vi "Test1_Network Connectivity.vi"(8 "error in":errorcluster, 10 "command line":string="ping -n 2 127.0.0.1", 11 "Sequence Context In":refnum<k7>) -> (0 "error out":errorcluster, 3 "Return Packets(%)":i32=100)   [LabVIEW 2021]
doc: "You can use the System Exec VI to call command line utilities that return standard output to the command shell. You also can call interactive applications that you intend to launch using System Exec, but interact with using the UI of the executable."
uses:
  <vilib>/regexp/Match Regular Expression.xnode
panel:
  out "standard output":string="\r\nPinging 127.0.0.1 with 32 bytes of data:\r\nReply from 127.0.0.1: bytes=32 time<1ms TTL=128\r\nReply from 127.0.0.1: bytes=32 time<1ms TTL=128\r\n\r\nPing statistics for 127.0.0.1:\r\n    Packets: Sent = 2, Received = 2, Lost = 0 (0% loss),\r\nApproximate round trip times in milli-seconds:\r\n    Minimum = 0ms, Maximum = 0ms, Average = 0ms\r\n"
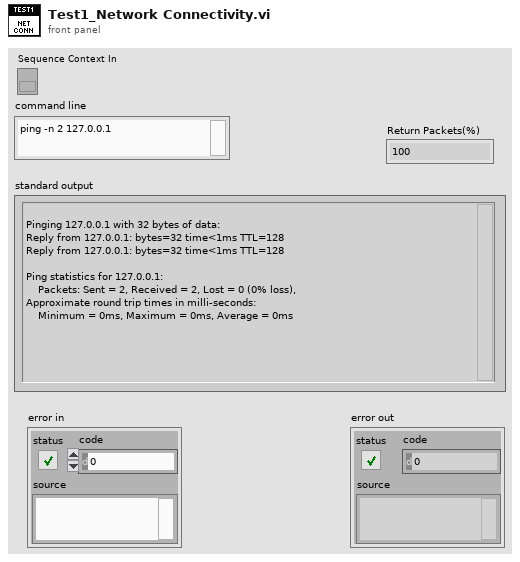
[diagram p1: front panel]
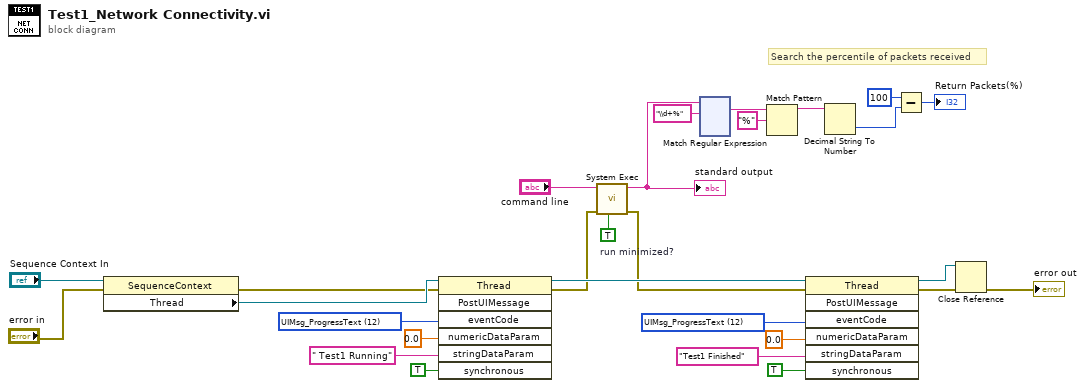
[diagram p0: block diagram]
diagram:
  w7 = 12 items=["UIMsg_BreakOnUserRequest"=1, "UIMsg_BreakOnBreakpoint"=2, "UIMsg_BreakOnRunTimeError"=3, "UIMsg_Trace"=4, "UIMsg_TerminatingExecution"=5, "UIMsg_AbortingExecution"=6, "UIMsg_KillingExecutionThreads"=7, "UIMsg_EndExecution"=8, "UIMsg_ShutDownComplete"=9, "UIMsg_StartExecution"=10, "UIMsg_ProgressPercent"=11, "UIMsg_ProgressText"=12, "UIMsg_StartInteractiveExecution"=13, "UIMsg_EndInteractiveExecution"=14, "UIMsg_TerminatingInteractiveExecution"=15, "UIMsg_TerminationCancelled"=16, "UIMsg_ResumeFromBreak"=17, "UIMsg_StartFileExecution"=18, "UIMsg_EndFileExecution"=19, "UIMsg_ShutDownCancelled"=20, "UIMsg_LocalizationSettingChanged"=21, "UIMsg_OpenWindows"=22, "UIMsg_TileWindows"=23, "UIMsg_CascadeWindows"=24, "UIMsg_ReportChanged"=25, "UIMsg_CloseWindows"=26, "UIMsg_RefreshWindows"=27, "UIMsg_ClientFileChanged"=28, "UIMsg_DisplayReport"=29, "UIMsg_ModelState_Initializing"=30, "UIMsg_ModelState_Waiting"=31, "UIMsg_ModelState_Identified"=32, "UIMsg_ModelState_BeginTesting"=33, "UIMsg_ModelState_TestingComplete"=34, "UIMsg_ModelState_PostProcessingComplete"=35, "UIMsg_ModelState_EnabledStateSet"=36, "UIMsg_ReportLocationChanged"=37, "UIMsg_GotoLocation"=38, "UIMsg_PushUndoItem"=39, "UIMsg_OutputMessages"=40, "UIMsg_TypePaletteFileListChanged"=41, "UIMsg_NonTerminatableThreadsArePreventingTermination"=42, "UIMsg_ModelState_PostProcessing"=43, "UIMsg_ReportCollectionChanged"=44, "UIMsg_RuntimeError"=45, "UIMsg_UserMessageBase"=10000] ("eventCode")
  w14 = 12 items=["UIMsg_BreakOnUserRequest"=1, "UIMsg_BreakOnBreakpoint"=2, "UIMsg_BreakOnRunTimeError"=3, "UIMsg_Trace"=4, "UIMsg_TerminatingExecution"=5, "UIMsg_AbortingExecution"=6, "UIMsg_KillingExecutionThreads"=7, "UIMsg_EndExecution"=8, "UIMsg_ShutDownComplete"=9, "UIMsg_StartExecution"=10, "UIMsg_ProgressPercent"=11, "UIMsg_ProgressText"=12, "UIMsg_StartInteractiveExecution"=13, "UIMsg_EndInteractiveExecution"=14, "UIMsg_TerminatingInteractiveExecution"=15, "UIMsg_TerminationCancelled"=16, "UIMsg_ResumeFromBreak"=17, "UIMsg_StartFileExecution"=18, "UIMsg_EndFileExecution"=19, "UIMsg_ShutDownCancelled"=20, "UIMsg_LocalizationSettingChanged"=21, "UIMsg_OpenWindows"=22, "UIMsg_TileWindows"=23, "UIMsg_CascadeWindows"=24, "UIMsg_ReportChanged"=25, "UIMsg_CloseWindows"=26, "UIMsg_RefreshWindows"=27, "UIMsg_ClientFileChanged"=28, "UIMsg_DisplayReport"=29, "UIMsg_ModelState_Initializing"=30, "UIMsg_ModelState_Waiting"=31, "UIMsg_ModelState_Identified"=32, "UIMsg_ModelState_BeginTesting"=33, "UIMsg_ModelState_TestingComplete"=34, "UIMsg_ModelState_PostProcessingComplete"=35, "UIMsg_ModelState_EnabledStateSet"=36, "UIMsg_ReportLocationChanged"=37, "UIMsg_GotoLocation"=38, "UIMsg_PushUndoItem"=39, "UIMsg_OutputMessages"=40, "UIMsg_TypePaletteFileListChanged"=41, "UIMsg_NonTerminatableThreadsArePreventingTermination"=42, "UIMsg_ModelState_PostProcessing"=43, "UIMsg_ReportCollectionChanged"=44, "UIMsg_RuntimeError"=45, "UIMsg_UserMessageBase"=10000] ("eventCode")
  w28 = TRUE  # run minimized?
  # "Search the percentile of packets received"
  n1 = property class="SequenceContext"(reference="Sequence Context In", error in="error in") -> (error out=w15:errorcluster, "Thread"=w16:refnum<k7>)  [unwired: 1 out]
  n2 = invoke class="Thread" method="PostUIMessage"(reference=w16, error in=w15, "eventCode"=w14, "numericDataParam"=0.0, "stringDataParam"=" Test1 Running", "synchronous"=TRUE) -> (reference out=w10:refnum<k7>, error out=w9:errorcluster)  [unwired: 1 in, 5 out]
  n3 = call <vilib>:"System Exec.vi"("run minimized? (F)"=w28, "error in (no error)"=w9, "command line"="command line") -> ("error out"=w8:errorcluster, "standard output"=w27:string)  [unwired: 3 in, 4 out]
  "standard output" <- w27
  n4 = xnode "Match Regular Expression"("input string"=w27, "regular expression"="\\d+%") -> ("whole match"=w25:string)  [unwired: 4 in, 4 out]
  n5 = Match Pattern(string=w25, regular expression="%") -> (before substring=w23:string)  [unwired: 1 in, 3 out]
  n6 = invoke class="Thread" method="PostUIMessage"(reference=w10, error in=w8, "eventCode"=w7, "numericDataParam"=0.0, "stringDataParam"="Test1 Finished", "synchronous"=TRUE) -> (reference out=w2:refnum<k7>, error out=w3:errorcluster)  [unwired: 1 in, 5 out]
  n7 = Decimal String To Number(string=w23) -> (number=w21:i32)  [unwired: 2 in, 1 out]
  n8 = Subtract(x=100, y=w21) -> (x-y=→"Return Packets(%)":i32)
  n9 = Close Reference(reference=w2, error in (no error)=w3) -> (error out=→"error out":errorcluster)
